vi "_CSMObj-Enqueue Cross-Module Message.vi"(8 "Error in":errorcluster caption="Error in (no error)", 9 "High Priority?(F)":bool, 10 "Data":T1, 11 "CSMQ in":T4={"Requested Name"="", "Module Name"="", "Mode"=enum."Stand Alone", "Queue"=refnum, "CSM-Data"=refnum, "User Event"=refnum, "Status Change Event"=refnum, "Allowed Messages"=[], "Mode-Data"=refnum, "Group Name"="", "Exit Event"=refnum}) -> (0 "Error out":errorcluster, 3 "CSMQ out":T4={"Requested Name"="", "Module Name"="", "Mode"=enum."Stand Alone", "Queue"=refnum, "CSM-Data"=refnum, "User Event"=refnum, "Status Change Event"=refnum, "Allowed Messages"=[], "Mode-Data"=refnum, "Group Name"="", "Exit Event"=refnum})   [LabVIEW 2020, in "Communicable State Machine.lvlib"]
uses:
  Communicable State Machine.lvlib
  _CSMObj.ctl
  Priority Queue.lvclass
  _CSM_MODE.ctl
  _CSMObj-Data.ctl
  _CSM Status Change Event Data.ctl
  _CSMObj-ModeData.ctl
  _Cross CSM State Data.ctl
  _CSM_MSG_TYPE.ctl
  _Cross CSM State Response.ctl
  _CSM_Response Source Message.ctl
  Priority Queue.lvclass/Priority Queue.ctl
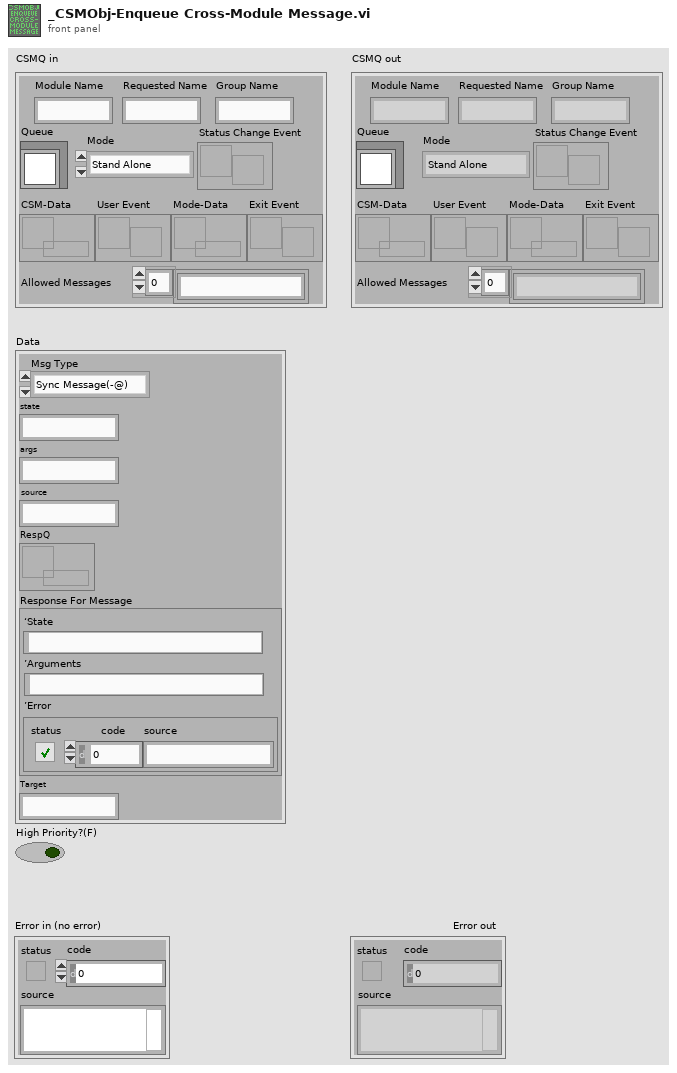
[diagram p1: front panel]
types:
  T1 = typedef "Communicable State Machine.lvlib/_Cross CSM State Data.ctl" = cluster{"Msg Type":T2, "state":string, "args":string, "source":string, "RespQ":refnum<queue>, "Response For Message":T3, "Target":string}
  T2 = typedef "Communicable State Machine.lvlib/_CSM_MSG_TYPE.ctl" = enum16{"Sync Message(-@)", "Async Message(->)", "Async without Response(->|)", "Async Response", "Broadcast(-><all>)", "Broadcast(-><status>)", "Broadcast(-><interrupt>)", "Append to JKISM States", "Append to JKISM States(High Priority)"}
  T3 = typedef "Communicable State Machine.lvlib/_CSM_Response Source Message.ctl" = cluster{"‘State":string, "’Arguments":string, "’Error":errorcluster}
  T4 = typedef "Communicable State Machine.lvlib/_CSMObj.ctl" = cluster{"Requested Name":string, "Module Name":string, "Mode":T5, "Queue":refnum<class "Priority Queue.lvclass">, "CSM-Data":refnum<data-value>, "User Event":refnum<user-event>, "Status Change Event":refnum<user-event>, "Allowed Messages":string[], "Mode-Data":refnum<data-value>, "Group Name":string, "Exit Event":refnum<user-event>}
  T5 = typedef "Communicable State Machine.lvlib/_CSM_MODE.ctl" = enum16{"Not Exist", "Stand Alone", "CSM", "Worker Agent", "Worker", "Chain", "Chain Node"}
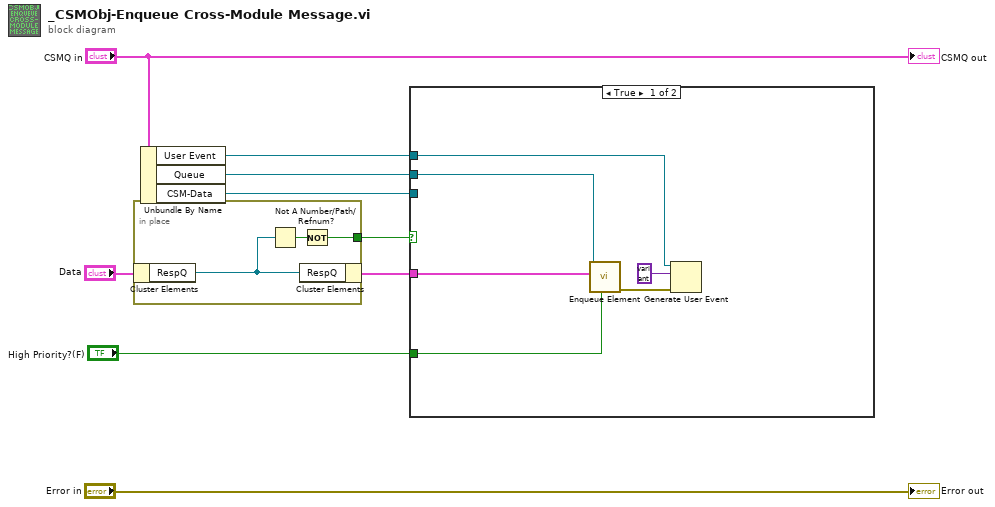
[diagram p0: block diagram]
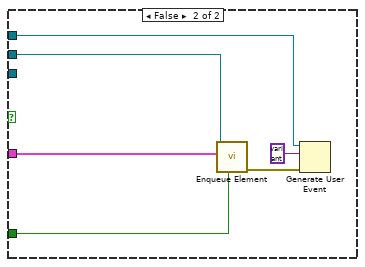
[diagram p2: hidden frame]
diagram:
  n1 = in-place {
    in-place-border: [w10] -> w5
    n2 = in-place-cluster #1("Data") -> ("RespQ"=w12:refnum<queue>)
    n3 = Not A Number/Path/Refnum?(number/path/refnum=w12) -> (NaN/Path/Refnum?=w11:bool)
    n4 = in-place-cluster #1("RespQ"=w12) -> (w6:T1)
    n5 = Not(x=w11) -> (.not. x?=w10:bool)
  }
  n6 = Unbundle By Name("CSMQ in") -> ("User Event"=w2:refnum<user-event>, "Queue"=w7:refnum<class "Priority Queue.lvclass">, "CSM-Data"=w4:refnum<data-value>)
  n7 = case shown="True" w5 {
    tunnel: w7 -> [w18 w24]
    tunnel: w6 -> [w17 w23]
    tunnel: w4 -> [_ _]
    tunnel: w2 -> [w16 w20]
    tunnel: "High Priority?(F)" -> [w15 w19]
    frame True {
      n8 = call "Enqueue Element.vi"("High Priority?(F)"=w15, "Cross JKI State Machine State"=w17, "Priority Queue"=w18) -> ("error out"=w14:errorcluster)  [unwired: 7 in, 1 out]
      n9 = Generate User Event(user event=w16, event data cluster=variant ("event data"), error in=w14) -> ()  [unwired: 1 in, 2 out]
    }
    frame False {
      n10 = call "Enqueue Element.vi"("High Priority?(F)"=w19, "Cross JKI State Machine State"=w23, "Priority Queue"=w24) -> ("error out"=w21:errorcluster)  [unwired: 7 in, 1 out]
      n11 = Generate User Event(user event=w20, event data cluster=variant ("event data"), error in=w21) -> ()  [unwired: 1 in, 2 out]
    }
  }
  "Error out" <- "Error in"
  "CSMQ out" <- "CSMQ in"
